vi "loads.vi"(8 "error in (no error)":errorcluster, 11 "path in":path) -> (0 "error out":errorcluster, 1 "dirty?":bool, 2 "sections":T1[](array[typedef]), 3 "path out":path)   [LabVIEW 2017, in "rpacini_toml.lvlib"]
uses:
  rpacini_toml.lvlib
  fg_section.ctl
  fg_row.ctl
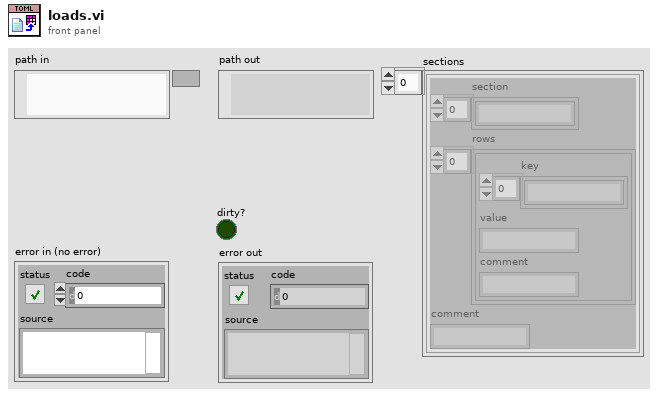
[diagram p1: front panel]
types:
  T1 = typedef "rpacini_toml.lvlib/fg_section.ctl" = cluster{"section":string[], "rows":T2[], "comment":string}
  T2 = typedef "rpacini_toml.lvlib/fg_row.ctl" = cluster{"key":string[], "value":string, "comment":string}
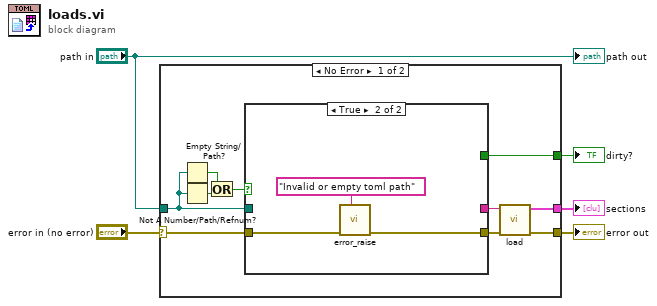
[diagram p0: block diagram]
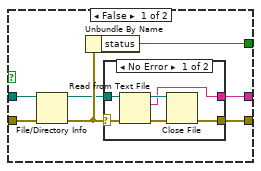
[diagram p2: hidden frame]
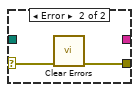
[diagram p3: hidden frame]
diagram:
  n1 = case shown="No Error" "error in (no error)" {
    selector: "error in (no error)" -> [w15 w34]
    tunnel: "path in" -> [w11 _]
    tunnel: [w12 w34] -> w3
    tunnel: [w7 _] -> w2
    tunnel: [w6 _] -> w1
    frame No Error {
      n2 = Empty String/Path?(string/path=w11) -> (empty?=w9:bool)
      n3 = Not A Number/Path/Refnum?(number/path/refnum=w11) -> (NaN/Path/Refnum?=w10:bool)
      n4 = Or(x=w9, y=w10) -> (x .or. y?=w8:bool)
      n5 = case shown="True" w8 {
        tunnel: [w22 _] -> w6
        tunnel: w15 -> [w21 w33]
        tunnel: [w18 w32] -> w14
        tunnel: [w17 _] -> w13
        tunnel: w11 -> [w16 _]
        frame False {
          n6 = File/Directory Info(path=w16, error in=w21) -> (path out=w19:path, error out=w20:errorcluster)  [unwired: 5 out]
          n7 = Unbundle By Name(w20) -> ("status"=w22:bool)
          n8 = case shown="No Error" w20 {
            selector: w20 -> [w26 w30]
            tunnel: w19 -> [w25 _]
            tunnel: [w24 w29] -> w18
            tunnel: [w23 _] -> w17
            frame No Error {
              n9 = Read from Text File(file (use dialog)=w25, error in=w26) -> (refnum out=w27:refnum<file>, text=w23:string, error out=w28:errorcluster)  [unwired: 2 in, 1 out]
              n10 = Close File(refnum=w27, error in=w28) -> (error out=w24:errorcluster)  [unwired: 1 out]
            }
            frame Error {
              n11 = call <vilib>:"Clear Errors.vi"("error in (no error)"=w30) -> ("error out"=w29:errorcluster)  [unwired: 5 in, 1 out]
            }
          }
        }
        frame True {
          n12 = call "error_raise.vi"("message"="Invalid or empty toml path", "error in (no error)"=w33) -> ("error out"=w32:errorcluster)  [unwired: 9 in]
        }
      }
      n13 = call "load.vi"("error in (no error)"=w14, "toml"=w13) -> ("error out"=w12:errorcluster, "sections"=w7:T1[])  [unwired: 8 in]
    }
    frame Error {
    }
  }
  "error out" <- w3
  "sections" <- w2
  "dirty?" <- w1
  "path out" <- "path in"
